vi "Create Name jettl Msg.vi"(6 "Name":string, 8 "error in":errorcluster, 9 "Name Library File Path":path, 10 "Active Project":refnum<vi>) -> (0 "error out":errorcluster, 2 "Name jettl Msg":T1)   [LabVIEW 2025, in "_Rescript.lvlib" / "Msg.lvlib" / "Msg.lvclass"]
uses:
  Msg.lvclass
  Name jettl Msg.ctl
  Msg.lvclass/Msg.ctl
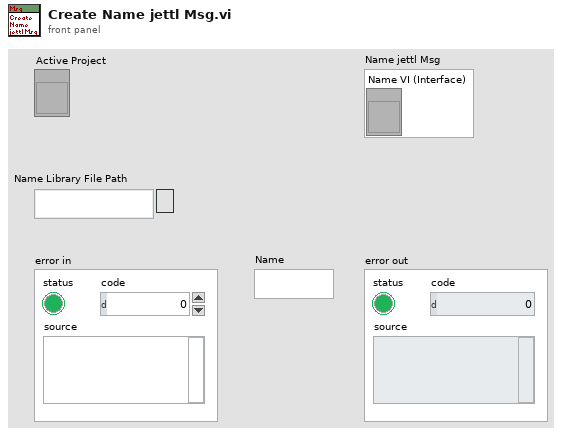
[diagram p1: front panel]
types:
  T1 = typedef "_Rescript.lvlib/Msg.lvlib/Msg.lvclass/Name jettl Msg.ctl" = cluster{"Name VI (Interface)":refnum<vi>}
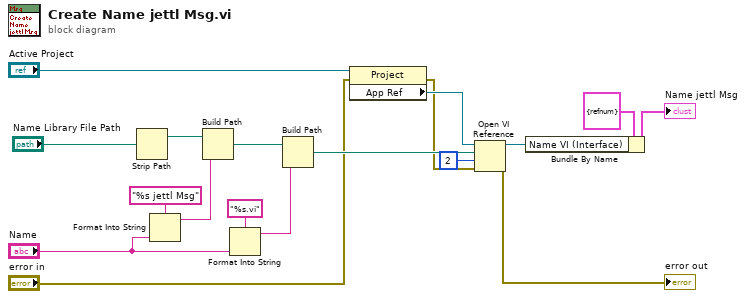
[diagram p0: block diagram]
diagram:
  n1 = Strip Path(path="Name Library File Path") -> (stripped path=w12:path)  [unwired: 1 out]
  n2 = Format Into String(format string="%s jettl Msg", "Name") -> (resulting string=w2:string)  [unwired: 2 in, 1 out]
  n3 = Build Path(base path=w12, name or relative path=w2) -> (appended path=w18:path)
  n4 = Format Into String(format string="%s.vi", "Name") -> (resulting string=w17:string)  [unwired: 2 in, 1 out]
  n5 = Build Path(base path=w18, name or relative path=w17) -> (appended path=w15:path)
  n6 = property class="Project"(reference="Active Project", error in="error in") -> (error out=w5:errorcluster, "App Ref"=w6:refnum<vi>)  [unwired: 1 out]
  n7 = Open VI Reference(application reference (local)=w6, vi path=w15, options=2, error in (no error)=w5) -> (vi reference=w9:refnum<vi>, error out=→"error out":errorcluster)  [unwired: 2 in]
  n8 = Bundle By Name(cluster=T1 {"Name VI (Interface)"=refnum} ("Name Refs"), "Name VI (Interface)"=w9) -> (→"Name jettl Msg":T1)
